vi "Write Currently Temperature.vi"(8 "error in (no error)":errorcluster, 10 "Currently Temperature":i16, 11 "Simulated_Cooler in":refnum<class "Simulated_Cooler.lvclass">) -> (0 "error out":errorcluster, 3 "Simulated_Cooler out":refnum<class "Simulated_Cooler.lvclass">)   [LabVIEW 2018, in "Simulated_Cooler.lvclass"]
uses:
  Simulated_Cooler.lvclass
  Simulated_Cooler.lvclass/Simulated_Cooler.ctl
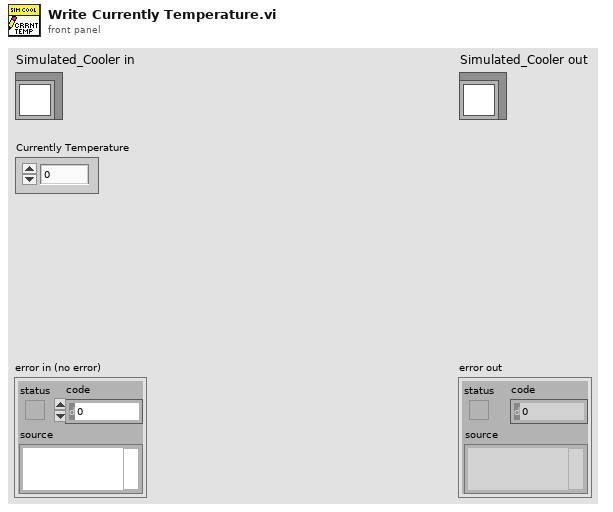
[diagram p1: front panel]
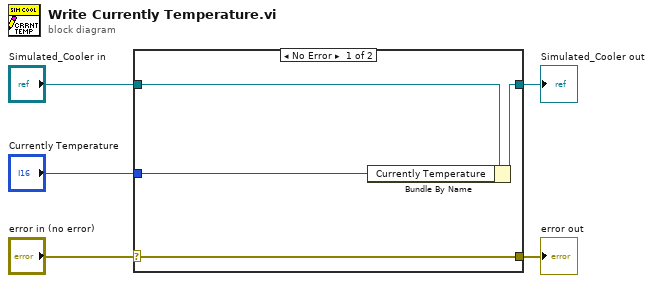
[diagram p0: block diagram]
diagram:
  n1 = case shown="No Error" "error in (no error)" {
    selector: "error in (no error)" -> [w9 w10]
    tunnel: [w9 w10] -> w4
    tunnel: [w7 w11] -> w2
    tunnel: "Simulated_Cooler in" -> [w8 w11]
    tunnel: "Currently Temperature" -> [w6 _]
    frame No Error {
      n2 = Bundle By Name(cluster=w8, "Currently Temperature"=w6) -> (w7:refnum<class "Simulated_Cooler.lvclass">)
    }
    frame Error {
    }
  }
  "error out" <- w4
  "Simulated_Cooler out" <- w2
